vi "pirate.vi"(2 "NXT/EV3":T1) -> (0 "NXT/EV3 2":T1)   [LabVIEW 2016]
uses:
  <vilib>/NXT/Subs/LVHSConnector.ctl
  <vilib>/NXT/LegoClasses/BrickReference/BrickReference.lvclass
  <vilib>/NXT/Dual Mode Library/Sound/PlayD.vi
  <vilib>/NXT/Dual Mode Library/Sound/PlayF.vi
  <vilib>/NXT/Dual Mode Library/Sound/PlayG.vi
  <vilib>/NXT/Dual Mode Library/Sound/PlayA.vi
  <vilib>/NXT/Dual Mode Library/Sound/PlayAsharp.vi
  <vilib>/NXT/Dual Mode Library/Sound/PlayC.vi
  <vilib>/NXT/Dual Mode Library/Waits/Wait_Num.vi
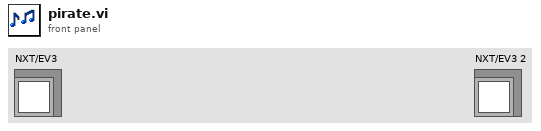
[diagram p1: front panel]
types:
  T1 = typedef "LVHSConnector.ctl" = refnum<class "BrickReference.lvclass">
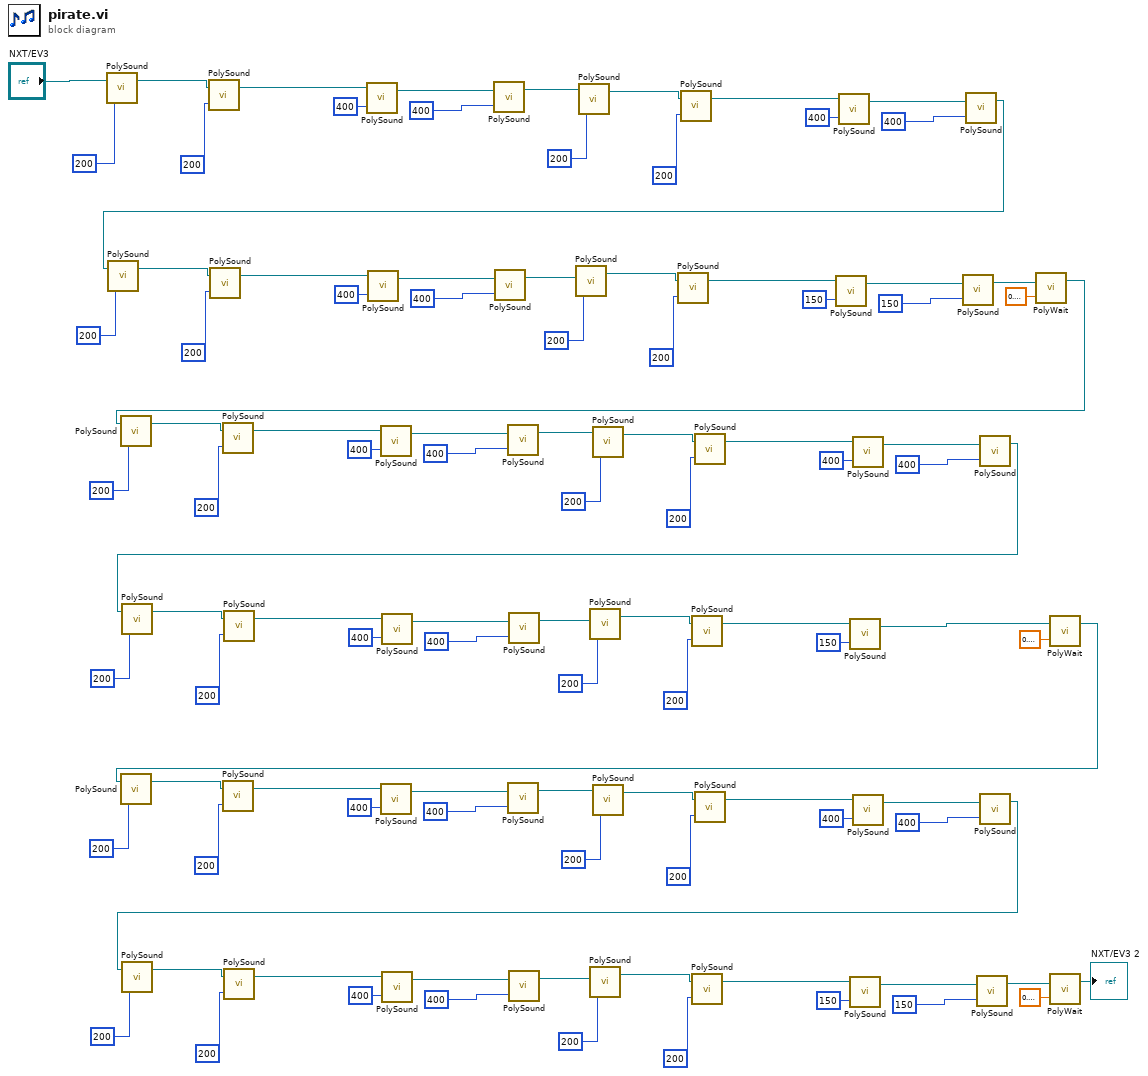
[diagram p0: block diagram]
diagram:
  n1 = call-poly <vilib>:"PolySound.vi"("Duration (500 ms)"=u16 200, "NXT/EV3"="NXT/EV3") -> ("NXT/EV3"=w97:T1)  [unwired: 2 in]
  n2 = call-poly <vilib>:"PolySound.vi"("Duration (500 ms)"=u16 200, "NXT/EV3"=w97) -> ("NXT/EV3"=w96:T1)  [unwired: 2 in]
  n3 = call-poly <vilib>:"PolySound.vi"("Duration (500 ms)"=u16 400, "NXT/EV3"=w96) -> ("NXT/EV3"=w95:T1)  [unwired: 2 in]
  n4 = call-poly <vilib>:"PolySound.vi"("Duration (500 ms)"=u16 400, "NXT/EV3"=w95) -> ("NXT/EV3"=w87:T1)  [unwired: 2 in]
  n5 = call-poly <vilib>:"PolySound.vi"("Duration (500 ms)"=u16 200, "NXT/EV3"=w87) -> ("NXT/EV3"=w90:T1)  [unwired: 2 in]
  n6 = call-poly <vilib>:"PolySound.vi"("Duration (500 ms)"=u16 200, "NXT/EV3"=w90) -> ("NXT/EV3"=w89:T1)  [unwired: 2 in]
  n7 = call-poly <vilib>:"PolySound.vi"("Duration (500 ms)"=u16 400, "NXT/EV3"=w89) -> ("NXT/EV3"=w88:T1)  [unwired: 2 in]
  n8 = call-poly <vilib>:"PolySound.vi"("Duration (500 ms)"=u16 400, "NXT/EV3"=w88) -> ("NXT/EV3"=w79:T1)  [unwired: 2 in]
  n9 = call-poly <vilib>:"PolySound.vi"("Duration (500 ms)"=u16 200, "NXT/EV3"=w79) -> ("NXT/EV3"=w82:T1)  [unwired: 2 in]
  n10 = call-poly <vilib>:"PolySound.vi"("Duration (500 ms)"=u16 200, "NXT/EV3"=w82) -> ("NXT/EV3"=w81:T1)  [unwired: 2 in]
  n11 = call-poly <vilib>:"PolySound.vi"("Duration (500 ms)"=u16 400, "NXT/EV3"=w81) -> ("NXT/EV3"=w80:T1)  [unwired: 2 in]
  n12 = call-poly <vilib>:"PolySound.vi"("Duration (500 ms)"=u16 400, "NXT/EV3"=w80) -> ("NXT/EV3"=w71:T1)  [unwired: 2 in]
  n13 = call-poly <vilib>:"PolySound.vi"("Duration (500 ms)"=u16 200, "NXT/EV3"=w71) -> ("NXT/EV3"=w74:T1)  [unwired: 2 in]
  n14 = call-poly <vilib>:"PolySound.vi"("Duration (500 ms)"=u16 200, "NXT/EV3"=w74) -> ("NXT/EV3"=w73:T1)  [unwired: 2 in]
  n15 = call-poly <vilib>:"PolySound.vi"("Duration (500 ms)"=u16 150, "NXT/EV3"=w73) -> ("NXT/EV3"=w72:T1)  [unwired: 2 in]
  n16 = call-poly <vilib>:"PolySound.vi"("Duration (500 ms)"=u16 150, "NXT/EV3"=w72) -> ("NXT/EV3"=w69:T1)  [unwired: 2 in]
  n17 = call-poly <vilib>:"PolyWait.vi"("Time (1 sec)"=sgl 0.4, "NXT/EV3"=w69) -> ("NXT/EV3"=w38:T1)  [unwired: 2 in]
  n18 = call-poly <vilib>:"PolySound.vi"("Duration (500 ms)"=u16 200, "NXT/EV3"=w38) -> ("NXT/EV3"=w64:T1)  [unwired: 2 in]
  n19 = call-poly <vilib>:"PolySound.vi"("Duration (500 ms)"=u16 200, "NXT/EV3"=w64) -> ("NXT/EV3"=w63:T1)  [unwired: 2 in]
  n20 = call-poly <vilib>:"PolySound.vi"("Duration (500 ms)"=u16 400, "NXT/EV3"=w63) -> ("NXT/EV3"=w62:T1)  [unwired: 2 in]
  n21 = call-poly <vilib>:"PolySound.vi"("Duration (500 ms)"=u16 400, "NXT/EV3"=w62) -> ("NXT/EV3"=w54:T1)  [unwired: 2 in]
  n22 = call-poly <vilib>:"PolySound.vi"("Duration (500 ms)"=u16 200, "NXT/EV3"=w54) -> ("NXT/EV3"=w57:T1)  [unwired: 2 in]
  n23 = call-poly <vilib>:"PolySound.vi"("Duration (500 ms)"=u16 200, "NXT/EV3"=w57) -> ("NXT/EV3"=w56:T1)  [unwired: 2 in]
  n24 = call-poly <vilib>:"PolySound.vi"("Duration (500 ms)"=u16 400, "NXT/EV3"=w56) -> ("NXT/EV3"=w55:T1)  [unwired: 2 in]
  n25 = call-poly <vilib>:"PolySound.vi"("Duration (500 ms)"=u16 400, "NXT/EV3"=w55) -> ("NXT/EV3"=w46:T1)  [unwired: 2 in]
  n26 = call-poly <vilib>:"PolySound.vi"("Duration (500 ms)"=u16 200, "NXT/EV3"=w46) -> ("NXT/EV3"=w49:T1)  [unwired: 2 in]
  n27 = call-poly <vilib>:"PolySound.vi"("Duration (500 ms)"=u16 200, "NXT/EV3"=w49) -> ("NXT/EV3"=w48:T1)  [unwired: 2 in]
  n28 = call-poly <vilib>:"PolySound.vi"("Duration (500 ms)"=u16 400, "NXT/EV3"=w48) -> ("NXT/EV3"=w47:T1)  [unwired: 2 in]
  n29 = call-poly <vilib>:"PolySound.vi"("Duration (500 ms)"=u16 400, "NXT/EV3"=w47) -> ("NXT/EV3"=w40:T1)  [unwired: 2 in]
  n30 = call-poly <vilib>:"PolySound.vi"("Duration (500 ms)"=u16 200, "NXT/EV3"=w40) -> ("NXT/EV3"=w42:T1)  [unwired: 2 in]
  n31 = call-poly <vilib>:"PolySound.vi"("Duration (500 ms)"=u16 200, "NXT/EV3"=w42) -> ("NXT/EV3"=w41:T1)  [unwired: 2 in]
  n32 = call-poly <vilib>:"PolySound.vi"("Duration (500 ms)"=u16 150, "NXT/EV3"=w41) -> ("NXT/EV3"=w37:T1)  [unwired: 2 in]
  n33 = call-poly <vilib>:"PolyWait.vi"("Time (1 sec)"=sgl 0.4, "NXT/EV3"=w37) -> ("NXT/EV3"=w3:T1)  [unwired: 2 in]
  n34 = call-poly <vilib>:"PolySound.vi"("Duration (500 ms)"=u16 200, "NXT/EV3"=w3) -> ("NXT/EV3"=w32:T1)  [unwired: 2 in]
  n35 = call-poly <vilib>:"PolySound.vi"("Duration (500 ms)"=u16 200, "NXT/EV3"=w32) -> ("NXT/EV3"=w31:T1)  [unwired: 2 in]
  n36 = call-poly <vilib>:"PolySound.vi"("Duration (500 ms)"=u16 400, "NXT/EV3"=w31) -> ("NXT/EV3"=w30:T1)  [unwired: 2 in]
  n37 = call-poly <vilib>:"PolySound.vi"("Duration (500 ms)"=u16 400, "NXT/EV3"=w30) -> ("NXT/EV3"=w22:T1)  [unwired: 2 in]
  n38 = call-poly <vilib>:"PolySound.vi"("Duration (500 ms)"=u16 200, "NXT/EV3"=w22) -> ("NXT/EV3"=w25:T1)  [unwired: 2 in]
  n39 = call-poly <vilib>:"PolySound.vi"("Duration (500 ms)"=u16 200, "NXT/EV3"=w25) -> ("NXT/EV3"=w24:T1)  [unwired: 2 in]
  n40 = call-poly <vilib>:"PolySound.vi"("Duration (500 ms)"=u16 400, "NXT/EV3"=w24) -> ("NXT/EV3"=w23:T1)  [unwired: 2 in]
  n41 = call-poly <vilib>:"PolySound.vi"("Duration (500 ms)"=u16 400, "NXT/EV3"=w23) -> ("NXT/EV3"=w14:T1)  [unwired: 2 in]
  n42 = call-poly <vilib>:"PolySound.vi"("Duration (500 ms)"=u16 200, "NXT/EV3"=w14) -> ("NXT/EV3"=w17:T1)  [unwired: 2 in]
  n43 = call-poly <vilib>:"PolySound.vi"("Duration (500 ms)"=u16 200, "NXT/EV3"=w17) -> ("NXT/EV3"=w16:T1)  [unwired: 2 in]
  n44 = call-poly <vilib>:"PolySound.vi"("Duration (500 ms)"=u16 400, "NXT/EV3"=w16) -> ("NXT/EV3"=w15:T1)  [unwired: 2 in]
  n45 = call-poly <vilib>:"PolySound.vi"("Duration (500 ms)"=u16 400, "NXT/EV3"=w15) -> ("NXT/EV3"=w6:T1)  [unwired: 2 in]
  n46 = call-poly <vilib>:"PolySound.vi"("Duration (500 ms)"=u16 200, "NXT/EV3"=w6) -> ("NXT/EV3"=w9:T1)  [unwired: 2 in]
  n47 = call-poly <vilib>:"PolySound.vi"("Duration (500 ms)"=u16 200, "NXT/EV3"=w9) -> ("NXT/EV3"=w8:T1)  [unwired: 2 in]
  n48 = call-poly <vilib>:"PolySound.vi"("Duration (500 ms)"=u16 150, "NXT/EV3"=w8) -> ("NXT/EV3"=w7:T1)  [unwired: 2 in]
  n49 = call-poly <vilib>:"PolySound.vi"("Duration (500 ms)"=u16 150, "NXT/EV3"=w7) -> ("NXT/EV3"=w4:T1)  [unwired: 2 in]
  n50 = call-poly <vilib>:"PolyWait.vi"("Time (1 sec)"=sgl 0.4, "NXT/EV3"=w4) -> ("NXT/EV3"=→"NXT/EV3 2":T1)  [unwired: 2 in]
